vi "IMAQDevice.constructor.vi"(0 "name":string, 2 "data in":string, 5 "error in (no error)":errorcluster) -> (14 "i ref out":refnum<vi>, 16 "data out":string, 19 "error out":errorcluster)   [LabVIEW 2014, in "IMAQDevice.lvlib"]
doc: "This is the constructor of a class.\n\nLicense Agreement for this software:\n\nCopyright (C)\nGesellschaft für Schwerionenforschung, GSI\nPlanckstr. 1\n64291 Darmstadt\nGermany\n\nContact: D.Beck@gsi.de \n\nThis program is free software; you can redistribute it and/or modify it under the terms of the \nGNU General Public License as published by the Free Software Foundation; either version 2 of \nthe license, or (at your option) any later version.\n\nThis program is distributed in the hope that it will be useful, but WITHOUT ANY WARRANTY; \nwithout even the implied warranty of MERCHANTABILITY or FITNESS FOR A PARTICULAR PURPOSE. See the GNU General License for more details (http://www.gnu.org).\n\nGesellschaft für Schwerionenforschung, GSI\nPlanckstr. 1, 64291 Darmstadt, Germany\nFor all questions and ideas contact: M.Richter@gsi.de, H.Brand@gsi.de or D.Beck@gsi.de.\nLast update: 16-JUN-2004"
uses:
  IMAQDevice.lvlib
  CSCore/CSApplicationBaseClasses/DeviceBase/DeviceBase.lvlib
  CSCore/CSSystem/CSSystemLib/CSSystemLib.lvlib
  CSCore/CSApplicationBaseClasses/DeviceBase/DeviceBase.myEventNames.ctl
  CSlibraries-extern/HGF/HGF_LVC/HGF_BaseClasses/HGF_Factory/HGF_Factory.lvclass
  CSlibraries-extern/HGF/HGF_LVC/HGF_IMAQ/HGF_IMAQDevice/HGF_IMAQDevice.lvclass
  CSlibraries-extern/HGF/HGF_LVC/HGF_IMAQ/HGF_IMAQFactory/HGF_IMAQFactory.lvclass
  CSlibraries-extern/DimLVEvent/LVDimInterface/LVDimInterface.lvlib
  CSCore/BaseProcess/BaseProcess.lvlib
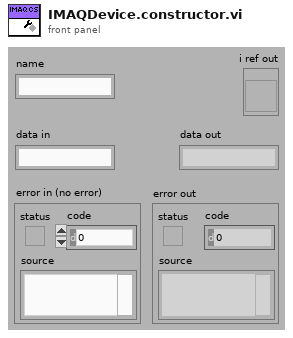
[diagram p1: front panel]
types:
  T1 = enum16{"SetAttribute", "GetAttribute", "CreateAttribute", "DestroyAttribute", "DestroyAllAtributes"}
  T2 = typedef "DeviceBase.lvlib/DeviceBase.myEventNames.ctl" = enum16{"lvmsg://Initialize", "lvmsg://Close", "lvmsg://Configure", "lvmsg://Reset", "lvmsg://IDQuery"}
  T3 = typedef "BaseProcess.lvlib/BaseProcess.i attribute.ctl" = cluster{"EventStatus":string, "EventError":i32, "PresetEvtWatchD":i32, "PresetPdcWatchD":i32, "EventTimeout":i32, "PeriodicInterval":i32, "Interface":string[], "Address":string[], "Special":string[], "PeriodicError":i32, "PeriodicStatus":string, "SuperProc":string, "Descriptors":T4[], "CaseRef":refnum<vi>, "PdcRef":refnum<vi>, "Thread Ref":refnum<vi>, "eventErrorID":i32, "eventStatusID":i32, "periodicErrorID":i32, "periodicStatusID":i32, "pdcCtrID":i32}
  T4 = typedef "BaseProcess.lvlib/BaseProcess.descriptor definition.ctl" = cluster{"selector":string, "descriptor":T5}
  T5 = typedef "BaseProcess.lvlib/BaseProcess.descriptor string definition.ctl" = string
  T6 = cluster{"Type":u32, "Version":u32, "Flags":u32, "SerialNumberHigh":u32, "SerialNumberLow":u32, "BusType":u32, "InterfaceName":string, "VendorName":string, "ModelName":string, "CameraFileName":string, "CameraAttributeURL":string}[]
  T7 = cluster{"1":cluster{i32, i32}, "2":cluster{i32, i32}, "3":cluster{i32, i32}, "4":cluster{i32, i32}}
  T8 = cluster{"1":cluster{dbl, dbl}, "2":cluster{dbl, dbl}, "3":cluster{dbl, dbl}, "4":cluster{dbl, dbl}}
  T9 = cluster{"Camera-Names":string[], "String":string}
  T10 = typedef "IMAQDevice.lvlib/IMAQDevice.i attribute.ctl" = cluster{"HGF_IMAQ.lvlib:HGF_IMAQDevice.lvclass":refnum<class "HGF_IMAQDevice.lvclass">, "Image":T11, "TimeStampID":i32, "Image IDs":i32[], "NumberOfImagesID":i32, "JPEG?":bool, "JPEGID":i32, "JPEG_ImageID":i32, "TriggerModeID":i32, "OffsetFromLeft":i32, "OffsetFromTop":i32, "HorizontalPixelPerMm":dbl, "VerticalPixelPerMm":dbl, "Grid":cluster{"1":cluster{i32, i32}, "2":cluster{i32, i32}, "3":cluster{i32, i32}, "4":cluster{i32, i32}}, "GridR":cluster{"1":cluster{dbl, dbl}, "2":cluster{dbl, dbl}, "3":cluster{dbl, dbl}, "4":cluster{dbl, dbl}}, "CameraTypeID":i32, "CameraInfos":cluster{"Camera Name-Array":string[], "own Camera Type":string}, "TakeMeasurement?":bool, "TriggerArmedID":i32, "Mirroring":i16, "Rotation":dbl}
  T11 = typedef "IMAQ Image.ctl" = refnum<image>
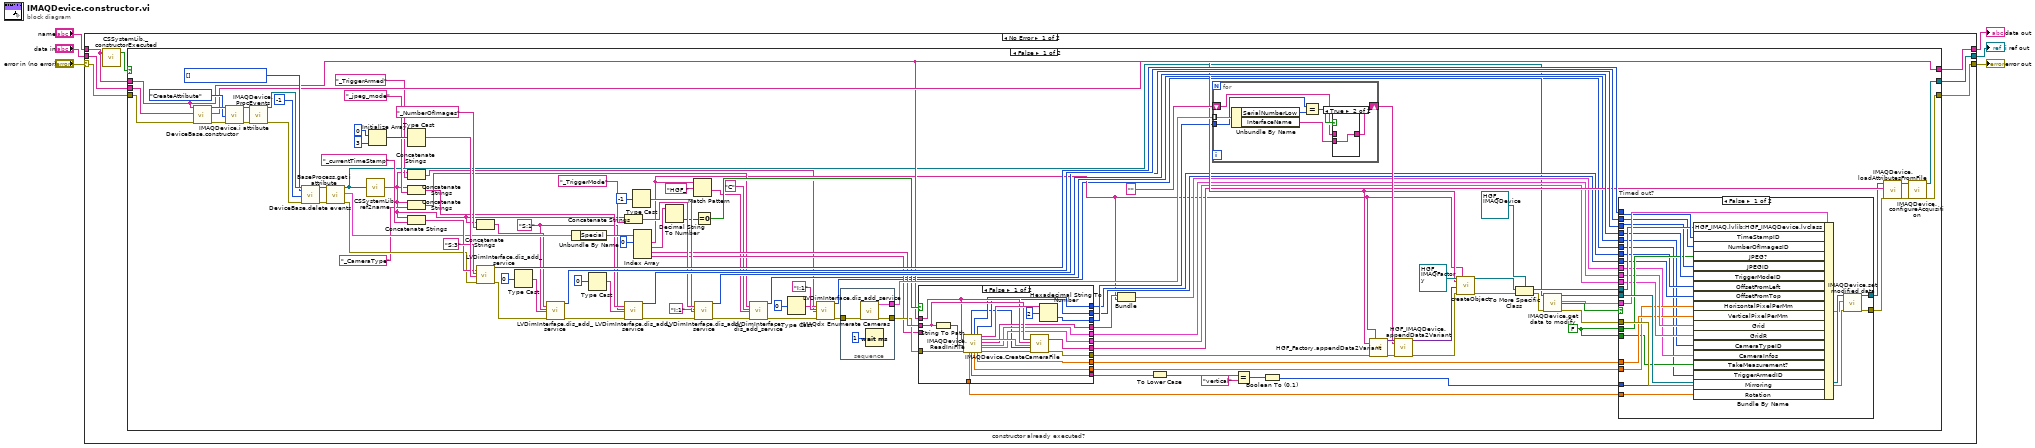
[diagram p0: block diagram]
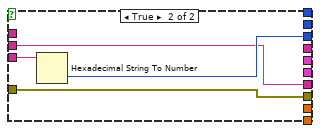
[diagram p2: hidden frame]
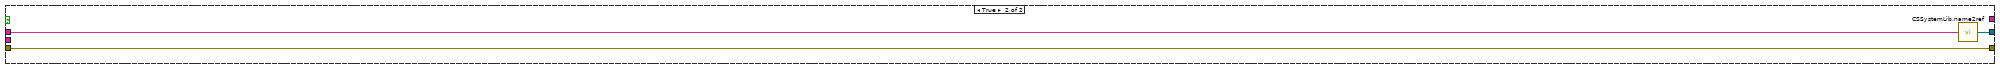
[diagram p5: hidden frame]
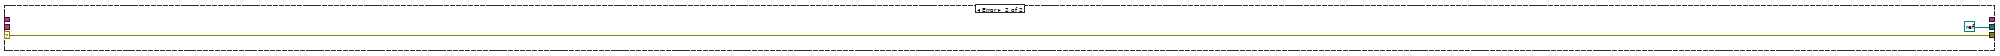
[diagram p6: hidden frame]
diagram:
  n1 = case shown="No Error" "error in (no error)" {
    selector: "error in (no error)" -> [w11 w193]
    tunnel: "name" -> [w10 _]
    tunnel: [w13 refnum<k0> refnum ("Not a Refnum Constant")] -> w5
    tunnel: [w12 w193] -> w4
    tunnel: "data in" -> [w8 _]
    tunnel: [w7 _] -> w1
    frame No Error {
      n2 = call "CSSystemLib._constructorExecuted.vi"("name"=w10) -> ("constructor executed?"=w9:bool)  [unwired: 18 in]
      n3 = case "constructor already executed?" shown="False" w9 {
        tunnel: w10 -> [w57 w192]
        tunnel: [w91 w191] -> w13
        tunnel: [w92 w190] -> w12
        tunnel: w11 -> [w120 w190]
        tunnel: w8 -> [w119 _]
        tunnel: [w114 _] -> w7
        frame False {
          w29 = FALSE
          w72 = "S:1" ("typeDescriptor")
          w116 = T2[] [] items=["lvmsg://Initialize", "lvmsg://Close", "lvmsg://Configure", "lvmsg://Reset", "lvmsg://IDQuery"] ("events")
          n4 = call "DeviceBase.constructor.vi"("name"=w57, "data in"=w119, "error in (no error)"=w120) -> ("i ref out"=w125:refnum<vi>, "data out"=w114:string, "error out"=w124:errorcluster)  [unwired: 14 in]
          n5 = call "IMAQDevice.i attribute.vi"("VI Refnum"=w125, "Action"=T1."CreateAttribute", "error in (no error)"=w124) -> ("VI Refnum out"=w122:refnum<vi>, "error out"=w121:errorcluster)  [unwired: 14 in, 1 out]
          n6 = call "IMAQDevice.ProcEvents.vi"("i ref in"=w122, "error in (no error)"=w121) -> ("i ref out"=w118:refnum<vi>, "error out"=w117:errorcluster)  [unwired: 16 in]
          n7 = call "DeviceBase.delete events.vi"("i ref in"=w118, "events"=w116, "ms timeout (10000)"=-1, "error in (no error)"=w117) -> ("i ref out"=w95:refnum<vi>, "error out"=w96:errorcluster)  [unwired: 13 in, 1 out]
          n8 = call "BaseProcess.get i attribute.vi"("i ref in"=w95, "error in (no error)"=w96) -> ("i ref out"=w38:refnum<vi>, "i attribute"=w94:T3, "error out"=w85:errorcluster)  [unwired: 15 in]
          n9 = call "CSSystemLib.ref2name.vi"("obj refnum"=w38) -> ("name"=w27:string)
          n10 = Initialize Array(i16 0 ("x"), 3 ("dimension size")) -> (w88:i16[])
          n11 = Type Cast(x=w88) -> (*(type *) &x=w105:string)  [unwired: 1 in]
          n12 = Concatenate Strings(w27, "_TriggerArmed" ("string")) -> (w24:string)
          n13 = Concatenate Strings(w27, "_jpeg_mode" ("string")) -> (w77:string)
          n14 = Concatenate Strings(w27, "_CameraType" ("string")) -> (w44:string)
          n15 = Concatenate Strings(w27, "_currentTimeStamp" ("string")) -> (w102:string)
          n16 = Concatenate Strings(w27, "_NumberOfImages" ("string")) -> (w82:string)
          n17 = call "LVDimInterface.dis_add_service.vi"("serviceName"=w102, "typeDescriptor"="S:3", "data"=w105, "error in (no error)"=w85) -> ("my_serviceID"=w101:i32, "error out"=w86:errorcluster)  [unwired: 14 in]
          n18 = Type Cast(x=i16 0) -> (*(type *) &x=w84:string)  [unwired: 1 in]
          n19 = call "LVDimInterface.dis_add_service.vi"("serviceName"=w82, "typeDescriptor"=w72, "data"=w84, "error in (no error)"=w86) -> ("my_serviceID"=w80:i32, "error out"=w76:errorcluster)  [unwired: 14 in]
          n20 = Unbundle By Name(w94) -> ("Special"=w79:string[])
          n21 = Type Cast(x=i16 0) -> (*(type *) &x=w74:string)  [unwired: 1 in]
          n22 = call "LVDimInterface.dis_add_service.vi"("serviceName"=w77, "typeDescriptor"=w72, "data"=w74, "error in (no error)"=w76) -> ("my_serviceID"=w75:i32, "error out"=w73:errorcluster)  [unwired: 14 in]
          n23 = Concatenate Strings(w27, "_TriggerMode" ("string")) -> (w70:string)
          n24 = Type Cast(x=-1) -> (*(type *) &x=w69:string)  [unwired: 1 in]
          n25 = Index Array(array=w79, index #1=0 ("index")) -> (element #1=w31:string, element #2=w61:string, element #3=w59:string, element #4=w56:string)  [unwired: 3 in]
          n26 = Decimal String To Number(string=w61) -> (number=w62:i32)  [unwired: 2 in, 1 out]
          n27 = Match Pattern(string=w31, regular expression="HGF_") -> (after substring=w32:string)  [unwired: 1 in, 3 out]
          n28 = call "LVDimInterface.dis_add_service.vi"("serviceName"=w70, "typeDescriptor"="I:1", "data"=w69, "error in (no error)"=w73) -> ("my_serviceID"=w67:i32, "error out"=w42:errorcluster)  [unwired: 14 in]
          n29 = Equal To 0?(x=w62) -> (x = 0?=w60:bool)
          n30 = call "LVDimInterface.dis_add_service.vi"("serviceName"=w44, "typeDescriptor"="C", "data"=w32, "error in (no error)"=w42) -> ("my_serviceID"=w46:i32, "error out"=w26:errorcluster)  [unwired: 14 in]
          n31 = Type Cast(x=0) -> (*(type *) &x=w21:string)  [unwired: 1 in]
          n32 = call "LVDimInterface.dis_add_service.vi"("serviceName"=w24, "typeDescriptor"="I:1", "data"=w21, "error in (no error)"=w26) -> ("my_serviceID"=w20:i32, "error out"=w25:errorcluster)  [unwired: 14 in]
          n33 = stacked-sequence {
            tunnel: [w129] -> w65
            tunnel: [w128] -> w58
            tunnel: w25 -> [w127]
            frame #0 {
              n34 = call <vilib>:"IMAQdx Enumerate Cameras.vi"("error in"=w127) -> ("error out"=w128:errorcluster, "Camera Information Array"=w129:T6)  [unwired: 9 in]
              n35 = Wait (ms)(milliseconds to wait=u32 1) -> ()  [unwired: 1 out]
            }
          }
          n36 = case shown="False" w60 {
            tunnel: w58 -> [w150 w152]
            tunnel: [w145 w152] -> w39
            tunnel: w57 -> [w143 _]
            tunnel: w59 -> [w144 w151]
            tunnel: w56 -> [_ w154]
            tunnel: [w147 w153] -> w55
            tunnel: [w141 w151] -> w54
            tunnel: [w140 _] -> w52
            tunnel: [w139 _] -> w51
            tunnel: [w138 _] -> w50
            tunnel: [w137 _] -> w49
            tunnel: [w136 _] -> w48
            tunnel: [w135 _] -> w47
            tunnel: [w134 _] -> w40
            tunnel: [w131 _] -> w19
            tunnel: [w130 _] -> w14
            frame False {
              n37 = String To Path(string=w144) -> (path=w149:path)
              n38 = call "IMAQDevice.ReadIniFile.vi"("ObjectName"=w143, "Path"=w149, "error in (no error)"=w150) -> ("Rotation"=w130:dbl, "TimeOut"=w132:i32, "Mirror"=w131:string, "OffsetFromLeft"=w135:i32, "HorizontalPixelPerMm"=w137:dbl, "OffsetFromTop"=w136:i32, "VerticalPixelPerMm"=w138:dbl, "Serial Number"=w148:string, "start sequence array"=w142:cluster{"Command":string, "Value":string}[], "Camera-Names"=w134:string[], "Grid"=w140:T7, "GridR"=w139:T8, "error out"=w146:errorcluster)  [unwired: 4 in]
              n39 = call "IMAQDevice.CreateCameraFile.vi"("Ini-File-Path"=w144, "Camera Name"=w143, "Attribute Array"=w142, "TimeOut"=w132, "error in"=w146) -> ("File Name"=w141:string, "error out"=w145:errorcluster)  [unwired: 13 in]
              n40 = Hexadecimal String To Number(string=w148, offset=2) -> (number=w147:u32)  [unwired: 1 in, 1 out]
            }
            frame True {
              n41 = Hexadecimal String To Number(string=w154) -> (number=w153:u32)  [unwired: 2 in, 1 out]
            }
          }
          n42 = Bundle("Camera-Names"=w40, "String"=w31) -> (w41:T9)  [unwired: 1 in]
          n43 = To Lower Case(string=w19) -> (all lower case string=w18:string)
          n44 = for {
            tunnel: w65 -> [w161] mode=indexing
            tunnel: w55 -> [w159]
            shift-right: [w155] -> w63
            shift-left: "" ("InterfaceName") -> [w156]
            n45 = Unbundle By Name(w161) -> ("SerialNumberLow"=w160:u32, "InterfaceName"=w157:string)
            n46 = Equal?(x=w159, y=w160) -> (x = y?=w158:bool)
            n47 = case shown="True" w158 {
              tunnel: w157 -> [_ w163]
              tunnel: w156 -> [w162 _]
              tunnel: [w162 w163] -> w155
              frame False {
              }
              frame True {
              }
            }
          }
          n48 = Equal?(x=w18, y="vertical") -> (x = y?=w16:bool)
          n49 = Boolean To (0,1)(Boolean=w16) -> (0, 1=w15:i16)
          n50 = call "HGF_Factory.appendData2Variant.vi"("objectName"=w57, "error in (no error)"=w39, "className"=w31) -> ("dup initData"=w109:variant, "error out"=w108:errorcluster)  [unwired: 15 in]
          n51 = call "HGF_IMAQDevice.appendData2Variant.vi"("initData"=w109, "cameraName"=w63, "error in (no error)"=w108) -> ("dup initData"=w110:variant, "error out"=w107:errorcluster)  [unwired: 15 in]
          n52 = call "createObject.vi"("HGF_Factory"=refnum<class "HGF_IMAQFactory.lvclass"> refnum ("HGF_IMAQ.lvlib:HGF_IMAQFactory.lvclass"), "objectName"=w57, "initializationData"=w110, "error in (no error)"=w107, "className"=w31) -> ("HGF_Object"=w98:refnum<class "HGF_Factory.lvclass">, "error out"=w97:errorcluster)  [unwired: 12 in, 1 out]
          n53 = To More Specific Class(target class=refnum<class "HGF_IMAQDevice.lvclass"> refnum ("HGF_IMAQ.lvlib:HGF_IMAQDevice.lvclass"), reference=w98, error in=w97) -> (specific class reference=w99:refnum<class "HGF_IMAQDevice.lvclass">, error out=w37:errorcluster)
          n54 = call "IMAQDevice.get data to modify.vi"("i ref in"=w38, "error in (no error)"=w37) -> ("i ref out"=w112:refnum<vi>, "i attribute"=w111:T10, "timed out"=w90:bool, "error out"=w113:errorcluster)  [unwired: 14 in]
          n55 = case "Timed out?" shown="False" w90 {
            tunnel: w113 -> [w187 w188]
            tunnel: w112 -> [w186 w189]
            tunnel: w111 -> [w185 _]
            tunnel: w101 -> [w183 _]
            tunnel: w99 -> [w182 _]
            tunnel: [w181 w188] -> w35
            tunnel: [w180 w189] -> w33
            tunnel: w80 -> [w179 _]
            tunnel: w75 -> [w178 _]
            tunnel: w67 -> [w177 _]
            tunnel: w29 -> [w176 _]
            tunnel: w52 -> [w175 _]
            tunnel: w51 -> [w174 _]
            tunnel: w50 -> [w173 _]
            tunnel: w49 -> [w172 _]
            tunnel: w48 -> [w171 _]
            tunnel: w47 -> [w170 _]
            tunnel: w46 -> [w169 _]
            tunnel: w41 -> [w168 _]
            tunnel: w29 -> [w167 _]
            tunnel: w20 -> [w166 _]
            tunnel: w15 -> [w165 _]
            tunnel: w14 -> [w164 _]
            frame False {
              n56 = Bundle By Name(cluster=w185, "HGF_IMAQ.lvlib:HGF_IMAQDevice.lvclass"=w182, "TimeStampID"=w183, "NumberOfImagesID"=w179, "JPEG?"=w176, "JPEGID"=w178, "TriggerModeID"=w177, "OffsetFromLeft"=w170, "OffsetFromTop"=w171, "HorizontalPixelPerMm"=w172, "VerticalPixelPerMm"=w173, "Grid"=w175, "GridR"=w174, "CameraTypeID"=w169, "CameraInfos"=w168, "TakeMeasurement?"=w167, "TriggerArmedID"=w166, "Mirroring"=w165, "Rotation"=w164) -> (w184:T10)
              n57 = call "IMAQDevice.set modified data.vi"("i ref in"=w186, "i attribute"=w184, "error in (no error)"=w187) -> ("i ref out"=w180:refnum<vi>, "error out"=w181:errorcluster)  [unwired: 15 in]
            }
            frame True {
            }
          }
          n58 = call "IMAQDevice.loadAttributesFromFile.vi"("i ref in"=w33, "File name"=w54, "error in (no error)"=w35) -> ("i ref out"=w34:refnum<vi>, "error out"=w36:errorcluster)  [unwired: 15 in]
          n59 = call "IMAQDevice.configureAcquisition.vi"("i ref in"=w34, "error in (no error)"=w36) -> ("i ref out"=w91:refnum<vi>, "error out"=w92:errorcluster)  [unwired: 16 in]
        }
        frame True {
          n60 = call "CSSystemLib.name2ref.vi"("name"=w192) -> ("obj refnum"=w191:refnum<vi>)
        }
      }
    }
    frame Error {
    }
  }
  "i ref out" <- w5
  "error out" <- w4
  "data out" <- w1
